vi "renk tanıma nesne takibi + foto çekme.vi"() -> ()   [LabVIEW 2017]
uses:
  <vilib>/userdefined/High Color/IMAQdx.ctl
  <vilib>/vision/driver/NI_Vision_Acquisition_Software.lvlib
  <vilib>/vision/NI_Vision_Development_Module.lvlib
panel:
  out "error out":errorcluster
  in  "foto çek":bool
  out "Kırmızı":bool
  out "Mavi":bool
  out "Yeşil":bool
  out "Color Spectrum":dbl[](array[numeric]) format="%.2f"
  in  "Color Sensitivity":u32(ring) items=["Low", "Medium", "High"]
  in  "stop":bool
  out "Image":T1(plugin-control)
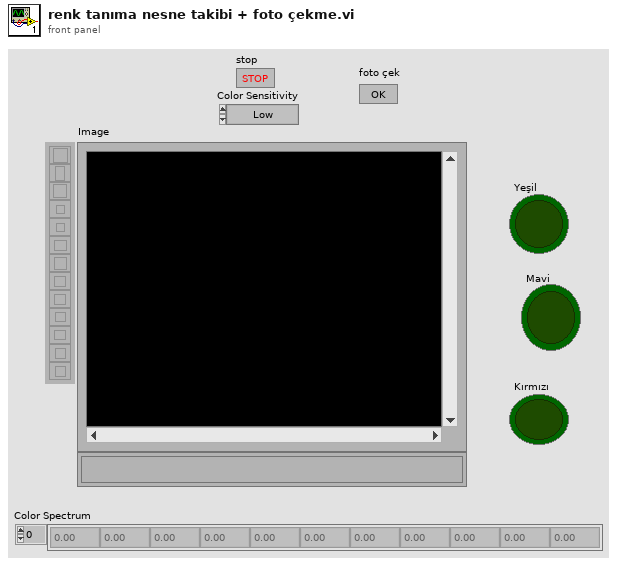
[diagram p1: front panel]
types:
  T1 = typedef "IMAQ Image.ctl" = refnum<image>
  T2 = typedef "IMAQdx.ctl" = refnum<k21>
  T3 = cluster{"Global Rectangle":i32[], "Contours":cluster{"Contour Type":u32, "ROI Type":u32, "Points":i32[]}[]}
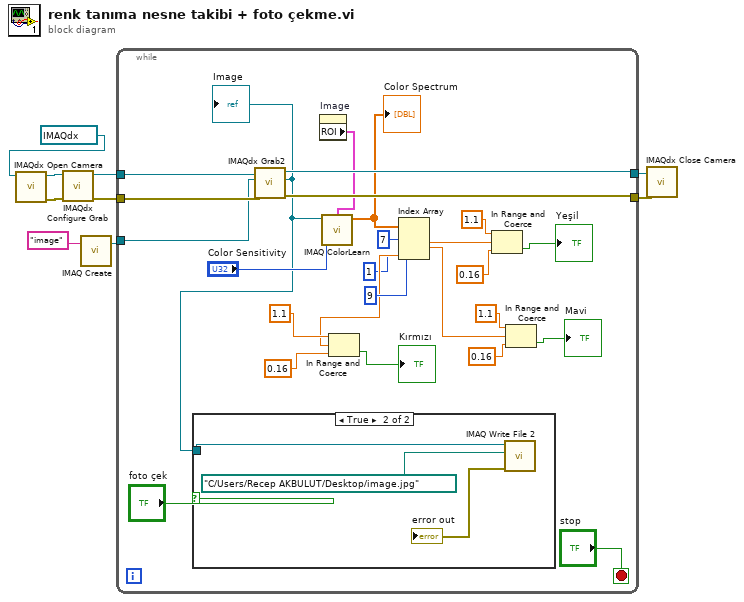
[diagram p0: block diagram]
diagram:
  n1 = call <vilib>:"IMAQdx Open Camera.vi"("Session In"=T2 "cam0") -> ("error out"=w8:errorcluster, "Session Out"=w9:T2)  [unwired: 9 in]
  n2 = call <vilib>:"IMAQdx Configure Grab.vi"("error in"=w8, "Session In"=w9) -> ("error out"=w5:errorcluster, "Session Out"=w6:T2)  [unwired: 8 in]
  n3 = call "IMAQ Create"("Image Name"="image") -> ("New Image"=w2:T1)  [unwired: 4 in, 1 out]
  n4 = while {
    tunnel: w6 -> [w35]
    tunnel: w5 -> [w34]
    tunnel: [w33] -> w4
    tunnel: [w32] -> w3
    tunnel: w2 -> [w31]
    stop <- "stop" stop-if-true
    n5 = call <vilib>:"IMAQdx Grab2.vi"("error in"=w34, "Image In"=w31, "Session In"=w35) -> ("error out"=w32:errorcluster, "Image Out"=w10:T1, "Session Out"=w33:T2)  [unwired: 5 in, 1 out]
    "Image" <- w10
    n6 = case shown="True" "foto çek" {
      tunnel: w10 -> [_ w38]
      frame False {
      }
      frame True {
        n7 = call-poly "IMAQ Write File 2"("File Path"=path "C:/Users/Recep AKBULUT/Desktop/image.jpg", "Image"=w38) -> ("error out"=→"error out":errorcluster)  [unwired: 8 in, 1 out]
      }
    }
    n8 = property on="Image" class="ImageControl"() -> ("ROI"=w28:T3)  [unwired: 2 in, 2 out]
    n9 = call "IMAQ ColorLearn"("ROI Descriptor"=w28, "Image"=w10, "Color Sensitivity"="Color Sensitivity") -> ("Color Spectrum"=w27:dbl[])  [unwired: 5 in, 1 out]
    "Color Spectrum" <- w27
    n10 = Index Array(array=w27, index #1=7 ("index"), index #2=9 ("index"), index #3=1 ("index")) -> (element #1=w23:dbl, element #2=w18:dbl, element #3=w14:dbl)
    n11 = In Range and Coerce(upper limit=1.1, x=w14, lower limit=0.16) -> (In Range?=→"Kırmızı":bool)  [unwired: 1 out]
    n12 = In Range and Coerce(upper limit=1.1, x=w23, lower limit=0.16) -> (In Range?=→"Yeşil":bool)  [unwired: 1 out]
    n13 = In Range and Coerce(upper limit=1.1, x=w18, lower limit=0.16) -> (In Range?=→"Mavi":bool)  [unwired: 1 out]
  }
  n14 = call <vilib>:"IMAQdx Close Camera.vi"("error in"=w3, "Session In"=w4) -> ()  [unwired: 9 in, 1 out]
